vi "Source DC Voltage.vi"(8 "error in (no error)":errorcluster, 10 "Params":variant, 11 "NI SMU in":refnum<class "NI SMU.lvclass">) -> (0 "error out":errorcluster, 3 "NI SMU out":refnum<class "NI SMU.lvclass">)   [LabVIEW 2020, in "NI SMU.lvlib" / "NI SMU.lvclass"]
uses:
  NI SMU.lvclass
  NI SMU.lvclass/NI SMU.ctl
  TypeDefs/DC voltage settings.ctl
  <instrlib>/niDCPower/nidcpower.llb/niDCPower Output Function.ctl
  <instrlib>/niDCPower/nidcpower.llb/niDCPower Source Mode.ctl
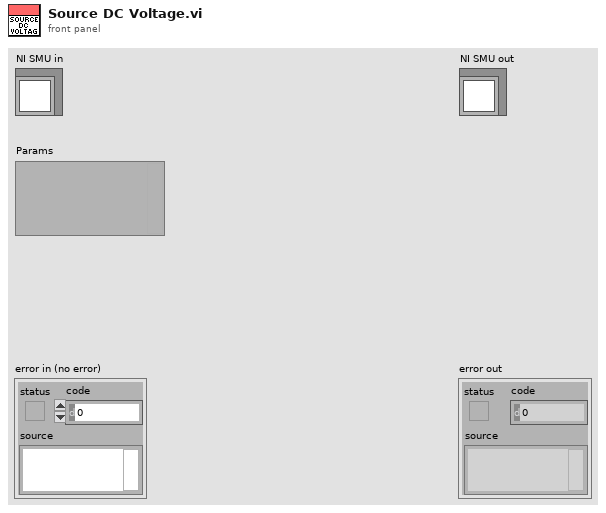
[diagram p1: front panel]
types:
  T1 = typedef "NI SMU.lvlib/NI SMU.lvclass/DC voltage settings.ctl" = cluster{"voltage level":dbl, "voltage level range":dbl, "current limit":dbl, "current limit range":dbl, "source delay":dbl}
  T2 = typedef "niDCPower Output Function.ctl" = i32
  T3 = typedef "niDCPower Source Mode.ctl" = i32
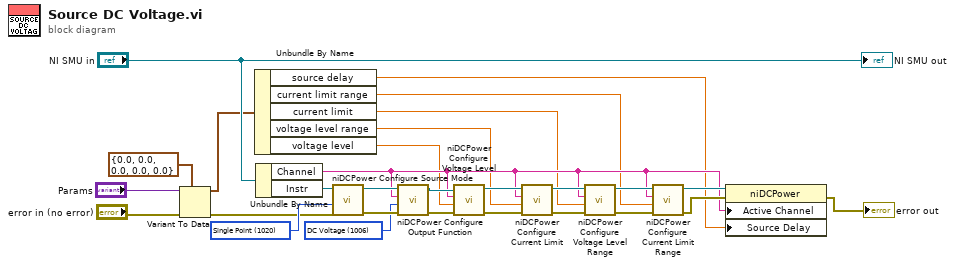
[diagram p0: block diagram]
diagram:
  w15 = T2 1006 items=["DC Voltage"=1006, "DC Current"=1007, "Pulse Voltage"=1049, "Pulse Current"=1050] ("output function")
  w24 = T3 1020 items=["Single Point"=1020, "Sequence"=1021] ("source mode")
  n1 = Variant To Data(error in="error in (no error)", type=T1 {"voltage level"=0.0, "voltage level range"=0.0, "current limit"=0.0, "current limit range"=0.0, "source delay"=0.0}, Variant="Params") -> (data=w6:T1, error out=w7:errorcluster)
  n2 = Unbundle By Name(w6) -> ("source delay"=w1:dbl, "current limit range"=w2:dbl, "current limit"=w3:dbl, "voltage level range"=w4:dbl, "voltage level"=w5:dbl)
  n3 = Unbundle By Name("NI SMU in") -> ("Channel"=w13:string, "Instr"=w12:refnum<k15>)
  n4 = call <instrlib>:"niDCPower Configure Source Mode.vi"("error in (no error)"=w7, "source mode"=w24, "instrument handle"=w12) -> ("error out"=w26:errorcluster, "instrument handle out"=w25:refnum<k15>)  [unwired: 7 out]
  n5 = call <instrlib>:"niDCPower Configure Output Function.vi"("error in (no error)"=w26, "output function"=w15, "channel name"=w13, "instrument handle"=w25) -> ("error out"=w16:errorcluster, "instrument handle out"=w17:refnum<k15>)  [unwired: 6 out]
  n6 = call <instrlib>:"niDCPower Configure Voltage Level.vi"("error in (no error)"=w16, "voltage level"=w5, "channel name"=w13, "instrument handle"=w17) -> ("error out"=w27:errorcluster, "instrument handle out"=w28:refnum<k15>)  [unwired: 6 out]
  n7 = call <instrlib>:"niDCPower Configure Current Limit.vi"("error in (no error)"=w27, "current limit"=w4, "channel name"=w13, "instrument handle"=w28) -> ("error out"=w23:errorcluster, "instrument handle out"=w22:refnum<k15>)  [unwired: 1 in, 5 out]
  n8 = call <instrlib>:"niDCPower Configure Voltage Level Range.vi"("error in (no error)"=w23, "voltage level range"=w3, "channel name"=w13, "instrument handle"=w22) -> ("error out"=w21:errorcluster, "instrument handle out"=w20:refnum<k15>)  [unwired: 6 out]
  n9 = call <instrlib>:"niDCPower Configure Current Limit Range.vi"("error in (no error)"=w21, "current limit range"=w2, "channel name"=w13, "instrument handle"=w20) -> ("error out"=w18:errorcluster, "instrument handle out"=w19:refnum<k15>)  [unwired: 6 out]
  n10 = property class="niDCPower"(reference=w19, error in=w18, "Active Channel"=w13, "Source Delay"=w1) -> (error out=→"error out":errorcluster)  [unwired: 1 out]
  "NI SMU out" <- "NI SMU in"
